vi "enterControl.vi"(8 "error in (no error)":errorcluster, 11 "Context in":refnum<class "Context.lvclass">) -> (0 "error out":errorcluster, 3 "Context out":refnum<class "Context.lvclass">)   [LabVIEW 2016, in "Context.lvclass"]
uses:
  Context.lvclass
  Context.lvclass/Context.ctl
  States/State/State.lvclass
  Model/Model.lvclass
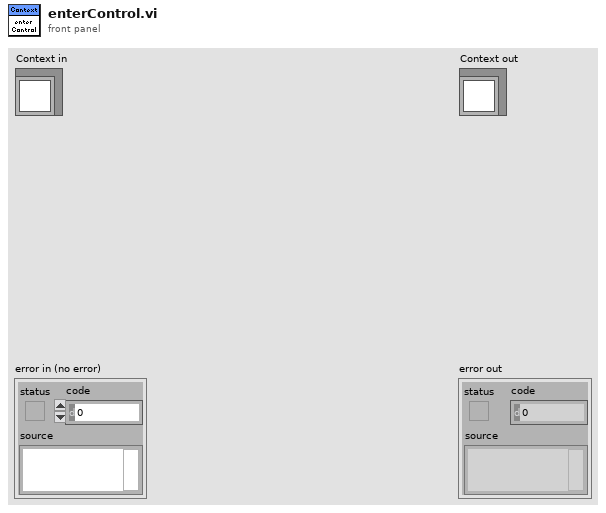
[diagram p1: front panel]
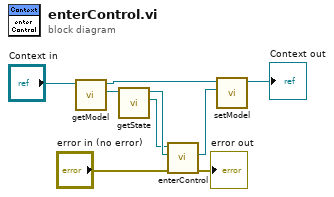
[diagram p0: block diagram]
diagram:
  n1 = call "getModel.vi"("Context in"="Context in") -> ("Model"=w2:refnum<class "Model.lvclass">, "Context out"=w4:refnum<class "Context.lvclass">)  [unwired: 9 in]
  n2 = call "getState.vi"("Model in"=w2) -> ("State out"=w8:refnum<class "State.lvclass">, "Model out"=w9:refnum<class "Model.lvclass">)  [unwired: 8 in, 1 out]
  n3 = call-dynamic "enterControl.vi"("error in (no error)"="error in (no error)", "Model in"=w9, "State in"=w8) -> ("error out"=→"error out":errorcluster, "Model out"=w1:refnum<class "Model.lvclass">)  [unwired: 6 in, 1 out]
  n4 = call "setModel.vi"("Model"=w1, "Context in"=w4) -> ("Context out"=→"Context out":refnum<class "Context.lvclass">)  [unwired: 9 in]
